vi "WrtRecFile.vi"(0 "Syll Freqs":dbl[](array[numeric]), 1 "Catch":i32[](array[numeric]), 2 "Samples":i32, 3 "N Channel":i32, 4 "File Info":T1 {"Threshold" format="%.2f"; "T after" format="%.2f"; "T Before" format="%.2f"}, 5 "Catch":bool, 6 "AI Rate":sgl format="%.2f", 7 "Total Data Time":dbl, 8 "Trigger Times":dbl[](array[numeric]) format="%.2f", 9 "Input Path":path) -> ()   [LabVIEW 2019]
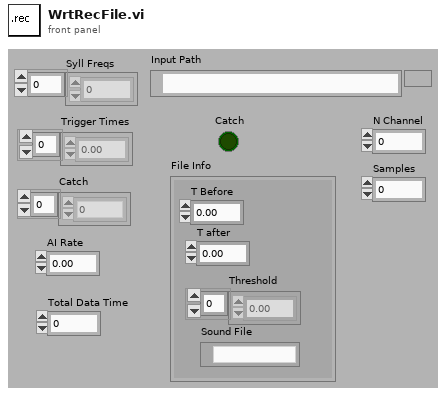
[diagram p1: front panel]
types:
  T1 = cluster{"T Before":dbl, "T after ":dbl, "Threshold":dbl[], "Sound File":path}
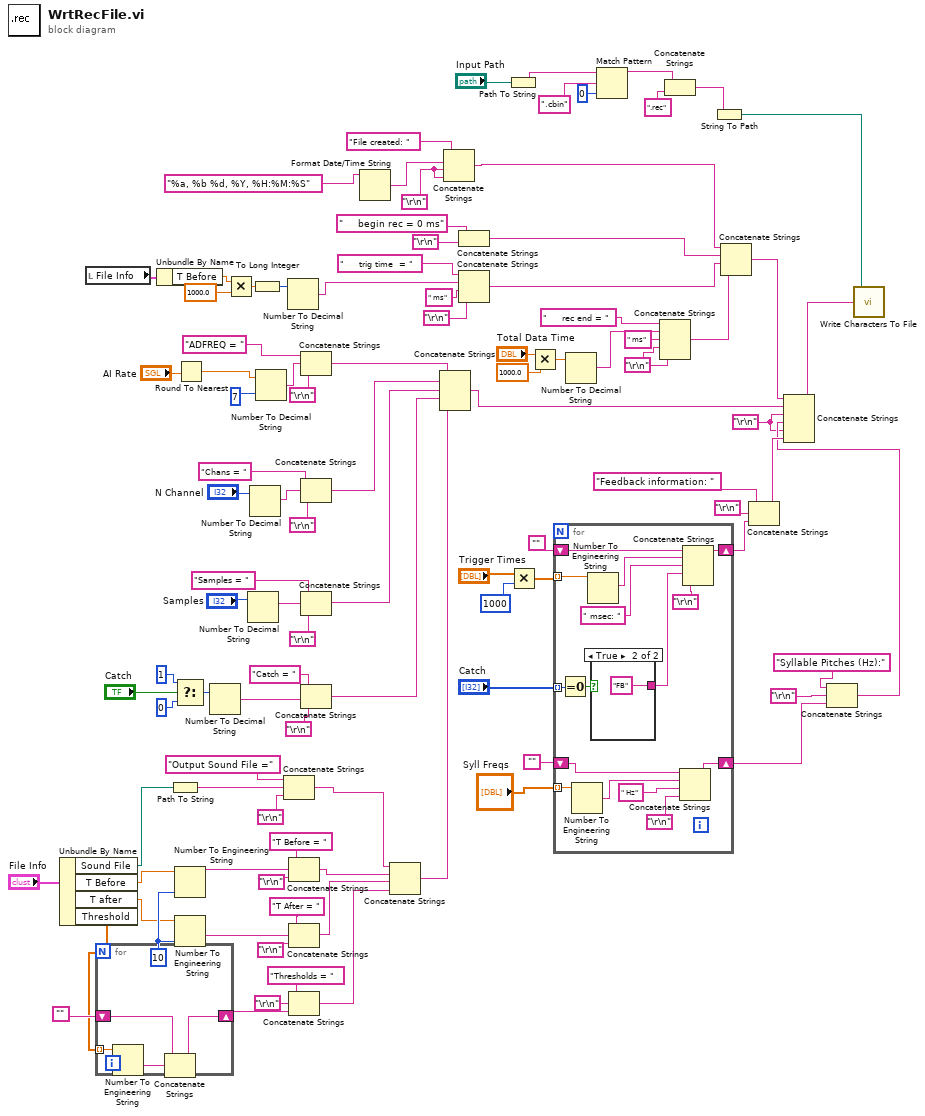
[diagram p0: block diagram]
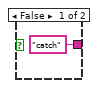
[diagram p2: hidden frame]
diagram:
  w3 = "\r\n"
  w32 = "\r\n"
  w50 = "\r\n"
  w61 = 10
  n1 = Unbundle By Name("File Info") -> ("Sound File"=w12:path, "T Before"=w20:dbl, "T after"=w19:dbl, "Threshold"=w18:dbl[])
  n2 = local read "File Info"() -> (w47:T1)
  n3 = for {
    shift-right: [w104] -> w58
    shift-left: "" -> [w105]
    tunnel: w18 -> [w103] mode=indexing
    n4 = Number To Engineering String(4:w103) -> (0:w107:string)  [unwired: 3 in]
    n5 = Concatenate Strings(w105, w107, "\r\n") -> (w104:string)
  }
  n6 = Unbundle By Name(w47) -> ("T Before"=w46:dbl)
  n7 = Path To String(path=w12) -> (string=w11:string)
  n8 = Select(t=1, s="Catch", f=0) -> (s? t:f=w76:i32)
  n9 = Number To Engineering String(2:w61, 4:w20) -> (0:w66:string)  [unwired: 2 in]
  n10 = Number To Engineering String(2:w61, 4:w19) -> (0:w65:string)  [unwired: 2 in]
  n11 = Round To Nearest(number="AI Rate") -> (nearest integer value=w52:sgl)
  n12 = Number To Decimal String(number=w76) -> (decimal integer string=w73:string)  [unwired: 1 in]
  n13 = Multiply(x=w46, y=1000.0) -> (x*y=w44:dbl)
  n14 = Number To Decimal String(number="Samples") -> (decimal integer string=w92:string)  [unwired: 1 in]
  n15 = Number To Decimal String(number="N Channel") -> (decimal integer string=w94:string)  [unwired: 1 in]
  n16 = To Long Integer(number=w44) -> (32bit integer=w43:i32)
  n17 = Number To Decimal String(number=w52, width (-)=i16 7 ("precision (6)")) -> (decimal integer string=w51:string)
  n18 = Concatenate Strings("Output Sound File =" ("string"), w11, "\r\n") -> (w10:string)
  n19 = Number To Decimal String(number=w43) -> (decimal integer string=w41:string)  [unwired: 1 in]
  n20 = Concatenate Strings("T Before = ", w66, "\r\n") -> (w15:string)
  n21 = Concatenate Strings("T After = ", w65, "\r\n") -> (w16:string)
  n22 = Concatenate Strings("Thresholds = ", "\r\n", w58) -> (w17:string)
  n23 = Concatenate Strings("ADFREQ = ", w51, "\r\n") -> (w91:string)
  n24 = Concatenate Strings("Chans = ", w94, "\r\n") -> (w90:string)
  n25 = Concatenate Strings("Samples = ", w92, "\r\n") -> (w89:string)
  n26 = Concatenate Strings("Catch = ", w73, "\r\n") -> (w72:string)
  n27 = Format Date/Time String(time format string (%c)="%a, %b %d, %Y, %H:%M:%S") -> (date/time string=w55:string)  [unwired: 2 in]
  n28 = Concatenate Strings(w10, w15, w16, w17) -> (w62:string)
  n29 = Concatenate Strings(w91, w90, w89, w72, w62) -> (w26:string)
  n30 = Concatenate Strings("File created: ", w55, w50, w50) -> (w31:string)
  n31 = Concatenate Strings("     begin rec = 0 ms", "\r\n") -> (w30:string)
  n32 = Concatenate Strings("     trig time  = ", w41, " ms", "\r\n") -> (w29:string)
  n33 = Path To String(path="Input Path") -> (string=w102:string)
  n34 = Multiply(x="Trigger Times", y=1000) -> (x*y=w21:dbl[])
  n35 = Multiply(x="Total Data Time", y=1000.0) -> (x*y=w35:dbl)
  n36 = for {
    tunnel: w21 -> [w122] mode=indexing
    shift-right: [w119] -> w2
    shift-left: "" -> [w121]
    tunnel: "Catch" -> [w116] mode=indexing
    shift-right: [w113] -> w1
    shift-left: "" -> [w112]
    tunnel: "Syll Freqs" -> [w109] mode=indexing
    n37 = Equal To 0?(x=w116) -> (x = 0?=w115:bool)
    n38 = Number To Engineering String(4:w109) -> (0:w114:string)  [unwired: 3 in]
    n39 = Number To Engineering String(4:w122) -> (0:w120:string)  [unwired: 3 in]
    n40 = case shown="True" w115 {
      tunnel: ["catch" "FB"] -> w110
      frame False {
      }
      frame True {
      }
    }
    n41 = Concatenate Strings(w112, w114, " Hz" ("string"), "\r\n") -> (w113:string)
    n42 = Concatenate Strings(w121, w120, " msec: ", w110, "\r\n") -> (w119:string)
  }
  n43 = Number To Decimal String(number=w35) -> (decimal integer string=w34:string)  [unwired: 1 in]
  n44 = Match Pattern(string=w102, regular expression=".cbin", offset (0)=0) -> (before substring=w88:string)  [unwired: 3 out]
  n45 = Concatenate Strings("     rec end = ", w34, " ms" ("string"), w32, w32) -> (w28:string)
  n46 = Concatenate Strings(w88, ".rec" ("Substring")) -> (w86:string)
  n47 = String To Path(string=w86) -> (path=w85:path)
  n48 = Concatenate Strings(w31, w30, w29, w28) -> (w27:string)
  n49 = Concatenate Strings("Feedback information: " ("Substring"), "\r\n", w2) -> (w5:string)
  n50 = Concatenate Strings("Syllable Pitches (Hz):" ("string"), "\r\n", w1) -> (w4:string)
  n51 = Concatenate Strings(w27, w26, w3, w4, w3, w5) -> (w71:string)
  n52 = call <vilib>:"Write Characters To File.vi"("character string"=w71, "file path (dialog if empty)"=w85) -> ()  [unwired: 3 in, 1 out]
